vi "Create Box.vi"(8 "Top":dbl, 9 "Bottom":dbl, 10 "Right":dbl, 11 "Left":dbl) -> (1 "Y":dbl[](array[numeric]), 2 "X":dbl[](array[numeric]), 3 "Box":cluster{dbl[], dbl[]})   [LabVIEW 2020]
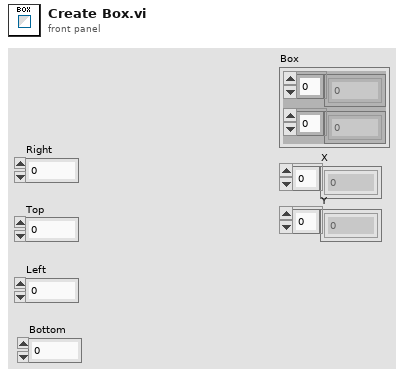
[diagram p1: front panel]
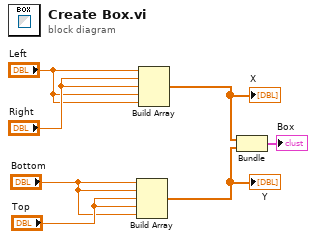
[diagram p0: block diagram]
diagram:
  n1 = Build Array("Bottom", "Bottom", "Top", "Top", "Bottom") -> (w2:dbl[])
  "Y" <- w2
  n2 = Build Array("Left", "Right", "Right", "Left", "Left") -> (w3:dbl[])
  "X" <- w3
  n3 = Bundle(w3, w2) -> (→"Box":cluster{dbl[], dbl[]})  [unwired: 1 in]
